vi "Load App Settings.vi"(8 "error in (no error)":errorcluster) -> (0 "error out":errorcluster)   [LabVIEW 2024, in "Data Base.lvlib"]
uses:
  Data Base.lvlib
  <vilib>/Utility/config.llb/Read Key (I32).vi
  Support/General Type Defs/Global Data.vi
  <vilib>/Utility/config.llb/Read Key (Boolean).vi
  <vilib>/Utility/config.llb/NI_LVConfig.lvlib
  Support/General Type Defs/General Type Definitions.lvlib
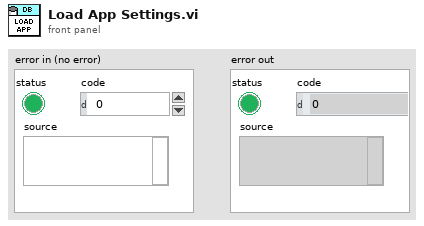
[diagram p1: front panel]
types:
  T1 = typedef "NI_LVConfig.lvlib/Config Data RefNum.ctl" = refnum<k1>
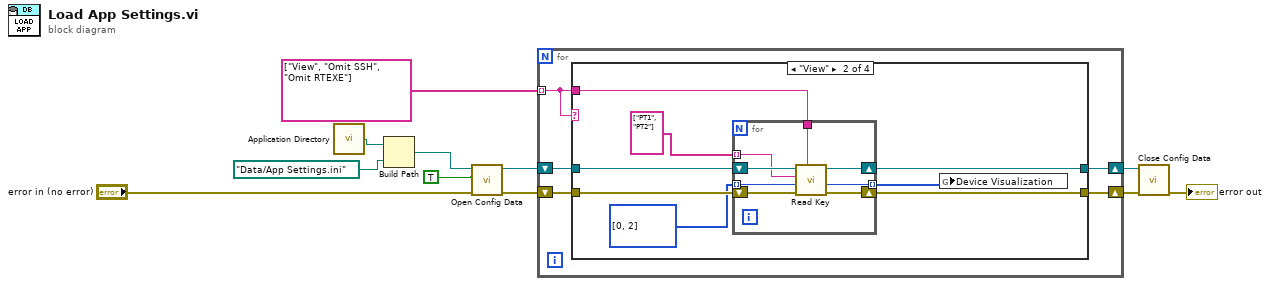
[diagram p0: block diagram]
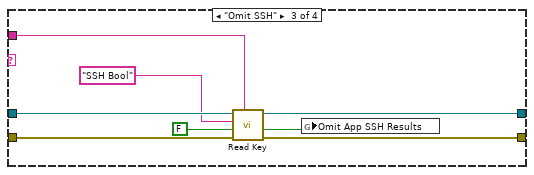
[diagram p3: hidden frame]
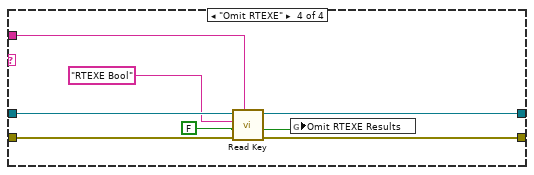
[diagram p4: hidden frame]
diagram:
  n1 = call <vilib>:"Application Directory.vi"() -> ("Application Directory"=w3:path)
  n2 = Build Path(base path=w3, name or relative path=path "Data/App Settings.ini") -> (appended path=w8:path)
  n3 = call <vilib>:"Open Config Data.vi"("error in (no error)"="error in (no error)", "create file if necessary (T)"=TRUE, "configuration file path"=w8) -> ("error out"=w5:errorcluster, "refnum"=w4:T1)  [unwired: 6 in, 1 out]
  n4 = for {
    shift-right: [w14] -> w6
    shift-left: w4 -> [w16]
    shift-right: [w13] -> w7
    shift-left: w5 -> [w15]
    tunnel: string[] ["View", "Omit SSH", "Omit RTEXE"] -> [w12] mode=indexing
    n5 = case shown="\"View\"" w12 {
      tunnel: w16 -> [w18 w26 w42 w50]
      tunnel: w15 -> [w17 w25 w41 w49]
      tunnel: [w18 w24 w40 w48] -> w14
      tunnel: [w17 w23 w39 w47] -> w13
      tunnel: w12 -> [_ w22 w38 w46]
      frame "", Default {
      }
      frame "View" {
        n6 = for {
          tunnel: w22 -> [w30]
          shift-right: [w32] -> w24
          shift-left: w26 -> [w34]
          shift-right: [w31] -> w23
          shift-left: w25 -> [w33]
          tunnel: string[] ["PT1", "PT2"] -> [w29] mode=indexing
          tunnel: [w28] -> w20 mode=indexing
          tunnel: i32[] [0, 2] -> [w27] mode=indexing
          n7 = call-poly <vilib>:"Read Key.vi"("section"=w30, "error in (no error)"=w33, "default value"=w27, "key"=w29, "refnum"=w34) -> ("error out"=w31:errorcluster, "value"=w28:i32, "refnum out"=w32:T1)  [unwired: 3 in, 1 out]
        }
        n8 = global write "Global Data.vi" "Device Visualization"(w20) -> ()
      }
      frame "Omit SSH" {
        n9 = call-poly <vilib>:"Read Key.vi"("section"=w38, "error in (no error)"=w41, "default value"=FALSE, "key"="SSH Bool", "refnum"=w42) -> ("error out"=w39:errorcluster, "value"=w36:bool, "refnum out"=w40:T1)  [unwired: 3 in, 1 out]
        n10 = global write "Global Data.vi" "Omit App SSH Results"(w36) -> ()
      }
      frame "Omit RTEXE" {
        n11 = call-poly <vilib>:"Read Key.vi"("section"=w46, "error in (no error)"=w49, "default value"=FALSE ("value"), "key"="RTEXE Bool", "refnum"=w50) -> ("error out"=w47:errorcluster, "value"=w43:bool, "refnum out"=w48:T1)  [unwired: 3 in, 1 out]
        n12 = global write "Global Data.vi" "Omit RTEXE Results"(w43) -> ()
      }
    }
  }
  n13 = call <vilib>:"Close Config Data.vi"("error in (no error)"=w7, "refnum"=w6) -> ("error out"=→"error out":errorcluster)  [unwired: 8 in, 1 out]
